vi "subElapsedTime.vi"(0 "Reset":bool, 1 "Elapsed Time Target":dbl=12.0 format="%0.8f", 2 "Set Start Time":dbl format="%0.2f", 3 "Auto Reset":bool=TRUE, 5 "error in (no error)":errorcluster) -> (9 "Elapsed TimeText":string, 11 "Present Text":string, 13 "Start Time Text":string, 14 "Time has Elapsed":bool, 15 "Elapsed Time":dbl format="%0.2f", 16 "Present":dbl format="%0.2f", 17 "Get Start Time":dbl format="%0.2f", 19 "error out":errorcluster)   [LabVIEW 2020]
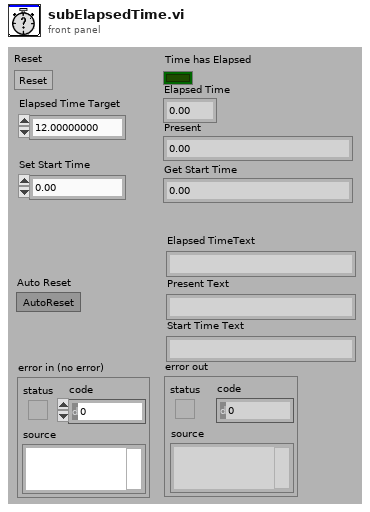
[diagram p1: front panel]
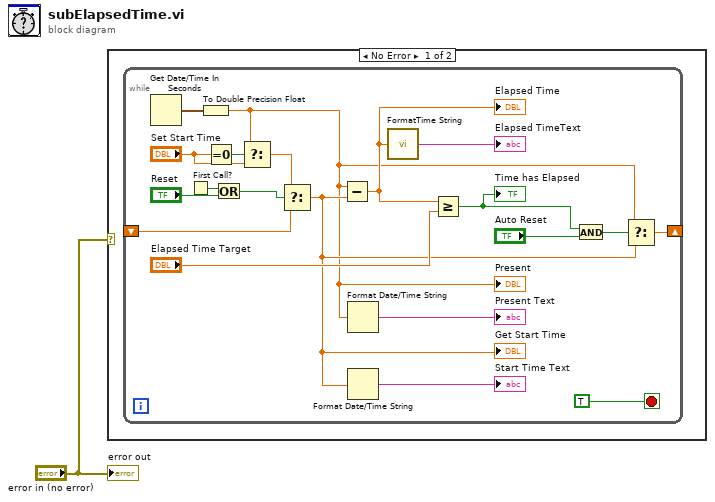
[diagram p0: block diagram]
diagram:
  n1 = case shown="No Error" "error in (no error)" {
    frame No Error {
      n2 = while {
        shift-right: [w6] -> _
        shift-left: _ -> [w15]
        stop <- TRUE stop-if-true
        n3 = Get Date/Time In Seconds() -> (seconds since 1Jan1904=w4:timestamp)
        n4 = First Call?() -> (First Call?: T/F=w18:bool)
        n5 = To Double Precision Float(number=w4) -> (double precision float=w3:dbl)
        "Present" <- w3
        n6 = Equal To 0?(x="Set Start Time") -> (x = 0?=w20:bool)
        n7 = Or(x=w18, y="Reset") -> (x .or. y?=w2:bool)
        n8 = Select(t=w3, s=w20, f="Set Start Time") -> (s? t:f=w21:dbl)
        n9 = Select(t=w21, s=w2, f=w15) -> (s? t:f=w7:dbl)
        "Get Start Time" <- w7
        n10 = Subtract(x=w3, y=w7) -> (x-y=w8:dbl)
        "Elapsed Time" <- w8
        n11 = Format Date/Time String(seconds (now)=w3) -> (date/time string=→"Present Text":string)  [unwired: 2 in]
        n12 = Format Date/Time String(seconds (now)=w7) -> (date/time string=→"Start Time Text":string)  [unwired: 2 in]
        n13 = call "FormatTime String.vi"("Numeric"=w8) -> ("Date/Time"=→"Elapsed TimeText":string)
        n14 = Greater Or Equal?(x=w8, y="Elapsed Time Target") -> (x >= y?=w13:bool)
        "Time has Elapsed" <- w13
        n15 = And(x=w13, y="Auto Reset") -> (x .and. y?=w5:bool)
        n16 = Select(t=w3, s=w5, f=w7) -> (s? t:f=w6:dbl)
      }
    }
    frame Error {
    }
  }
  "error out" <- "error in (no error)"
